vi "ScannedNodeSearch.vi"(6 "Location":T1, 8 "Previously Scanned Nodes":T4 {"Year" format="%02d"; "Patient Number" format="%03d"; "Node Number" format="%02d"}, 9 "Reset Node Count?":bool=TRUE, 10 "Auto Increment":bool, 11 "Searched Node":T2={"Patient Number"=0, "Node Set"="A", "Node Number"=0, "Tissue Type"=enum."Breast", "Tissue Location (Other)"="", "Node Classification"=enum."Whole Node", "Fresh?"=enum."Fresh?", "Year"=0} {"Year" format="%02d"; "Patient Number" format="%03d"; "Node Number" format="%02d"}) -> (3 "Next Node":T2={"Patient Number"=0, "Node Set"="A", "Node Number"=0, "Tissue Type"=enum."Breast", "Tissue Location (Other)"="", "Node Classification"=enum."Whole Node", "Fresh?"=enum."Fresh?", "Year"=0} {"Year" format="%02d"; "Patient Number" format="%03d"; "Node Number" format="%02d"})   [LabVIEW 2022 SP3]
uses:
  ScannedNodeArray.ctl
  LymphNodeInfo.ctl
  TissueTypeScan.ctl
  ScanningControl/-ScanSystem/Controls/location.ctl
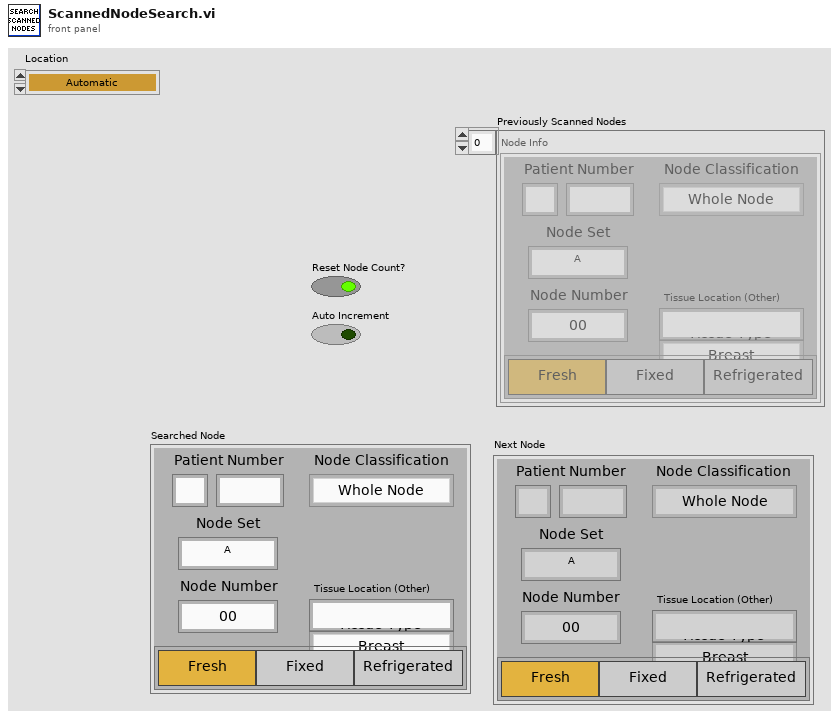
[diagram p1: front panel]
types:
  T1 = typedef "location.ctl" = enum16{"Automatic", "WCM Main", "Hawaii", "Columbia MM3000", "Columbia  NI System", "NYU", "RRI 2", "UHI Allen", "CUMC RT", "Chiba", "Stony Brook", "WCM Microscopy", "WCM Aeoretch", "WCM Optics Lab", "WCM Main 2Axis", "WCM Rotation", "WCM SAM SMAC", "SERI GP"}
  T2 = typedef "LymphNodeInfo.ctl" = cluster{"Patient Number":u32, "Node Set":string, "Node Number":u32, "Tissue Type":T3, "Tissue Location (Other)":string, "Node Classification":enum16{"Whole Node", "Piece A", "Piece B", "Piece C"}, "Fresh?":enum32{"Fresh?", "Fixed?", "Refrigerated?"}, "Year":u32}
  T3 = typedef "TissueTypeScan.ctl" = enum16{"Breast", "Gastric", "Stomach", "Rectal", "Colon", "Head & Neck", "Other"}
  T4 = typedef "ScannedNodeArray.ctl" = T2[]
  T5 = enum16{"Whole Node", "Piece A", "Piece B", "Piece C"}
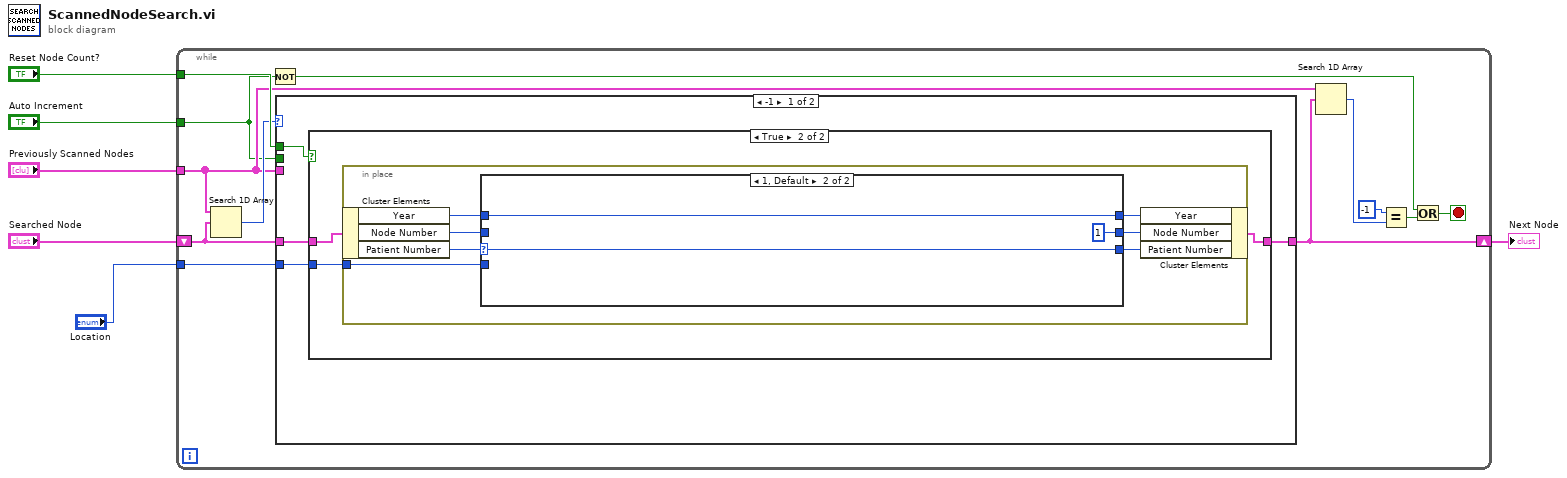
[diagram p0: block diagram]
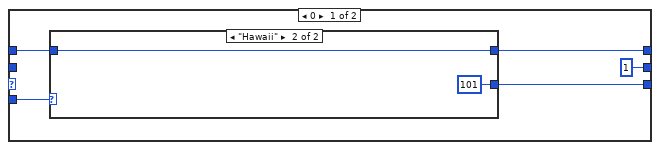
[diagram p3: hidden frame]
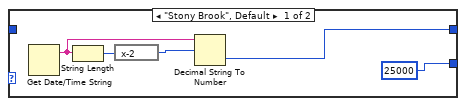
[diagram p4: hidden frame]
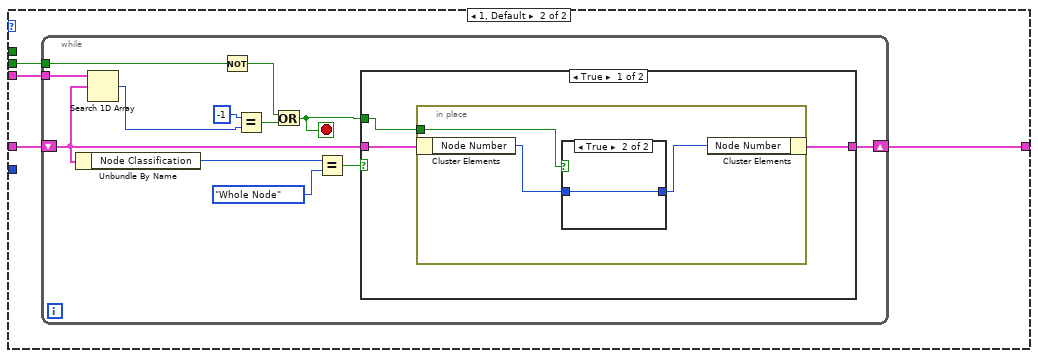
[diagram p5: hidden frame]
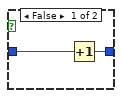
[diagram p6: hidden frame]
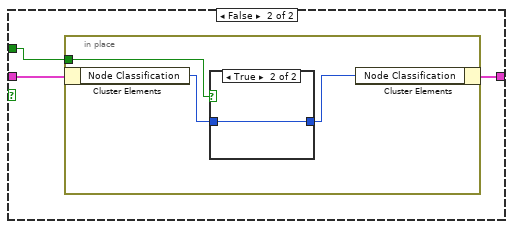
[diagram p7: hidden frame]
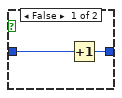
[diagram p8: hidden frame]
diagram:
  n1 = while {
    tunnel: "Reset Node Count?" -> [w17]
    tunnel: "Previously Scanned Nodes" -> [w13]
    tunnel: "Auto Increment" -> [w8]
    shift-right: [w14] -> w6
    shift-left: "Searched Node" -> [w18]
    tunnel: "Location" -> [w7]
    stop <- w9 stop-if-true
    n2 = Search 1D Array(1D array=w13, element=w18) -> (index of element=w15:i32)  [unwired: 1 in]
    n3 = Not(x=w8) -> (.not. x?=w11:bool)
    n4 = case shown="-1" w15 {
      tunnel: [w21 w51] -> w14
      tunnel: w18 -> [w22 w52]
      tunnel: w17 -> [w20 _]
      tunnel: w13 -> [_ w50]
      tunnel: w8 -> [_ w49]
      tunnel: w7 -> [w19 _]
      frame -1 {
        n5 = case shown="True" w20 {
          tunnel: w22 -> [w23 w26]
          tunnel: [w23 w25] -> w21
          tunnel: w19 -> [_ w24]
          frame False {
          }
          frame True {
            n6 = in-place {
              in-place-border: w24 -> [w29]
              n7 = in-place-cluster #1(w26) -> ("Year"=w27:u32, "Node Number"=w30:u32, "Patient Number"=w33:u32)
              n8 = case shown="1, Default" w33 {
                selector: w33 -> [_ w48]
                tunnel: [w38 w48] -> w32
                tunnel: [u32 1 ("Node Number") u32 1 ("Node Number")] -> w31
                tunnel: w30 -> [_ _]
                tunnel: w29 -> [w36 _]
                tunnel: [w35 w46] -> w28
                tunnel: w27 -> [w34 w46]
                frame 0 {
                  n9 = case shown="\"Hawaii\"" w36 {
                    tunnel: [u32 25000 ("y") u32 101] -> w38
                    tunnel: [w39 w44] -> w35
                    tunnel: w34 -> [_ w44]
                    frame "Stony Brook", Default {
                      n10 = Get Date/Time String() -> (date string=w42:string)  [unwired: 3 in, 1 out]
                      n11 = String Length(string=w42) -> (length=w43:i32)
                      n12 = expression code="x-2"(w43) -> (w41:i32)
                      n13 = Decimal String To Number(string=w42, offset=w41) -> (number=w39:i32)  [unwired: 1 in, 1 out]
                    }
                    frame "Hawaii" {
                    }
                  }
                }
                frame 1, Default {
                }
              }
              n14 = in-place-cluster #1("Year"=w28, "Node Number"=w31, "Patient Number"=w32) -> (w25:T2)
            }
          }
        }
      }
      frame 1, Default {
        n15 = while {
          shift-right: [w64] -> w51
          shift-left: w52 -> [w56]
          tunnel: w50 -> [w63]
          tunnel: w49 -> [w59]
          stop <- w57 stop-if-true
          n16 = Unbundle By Name(w56) -> ("Node Classification"=w53:T5)
          n17 = Search 1D Array(1D array=w63, element=w56) -> (index of element=w62:i32)  [unwired: 1 in]
          n18 = Not(x=w59) -> (.not. x?=w58:bool)
          n19 = Equal?(x=-1, y=w62) -> (x = y?=w60:bool)
          n20 = Or(x=w58, y=w60) -> (x .or. y?=w57:bool)
          n21 = Equal?(x=w53, y=T5."Whole Node") -> (x = y?=w55:bool)
          n22 = case shown="True" w55 {
            tunnel: [w67 w76] -> w64
            tunnel: w56 -> [w66 w75]
            tunnel: w57 -> [w65 w74]
            frame True {
              n23 = in-place {
                in-place-border: w65 -> [w68]
                n24 = in-place-cluster #2(w66) -> ("Node Number"=w70:u32)
                n25 = case shown="True" w68 {
                  tunnel: w70 -> [w72 w73]
                  tunnel: [w71 w73] -> w69
                  frame False {
                    n26 = Increment(x=w72) -> (x+1=w71:u32)
                  }
                  frame True {
                  }
                }
                n27 = in-place-cluster #2("Node Number"=w69) -> (w67:T2)
              }
            }
            frame False {
              n28 = in-place {
                in-place-border: w74 -> [w77]
                n29 = in-place-cluster #3(w75) -> ("Node Classification"=w79:T5)
                n30 = case shown="True" w77 {
                  tunnel: w79 -> [w81 w82]
                  tunnel: [w80 w82] -> w78
                  frame False {
                    n31 = Increment(x=w81) -> (x+1=w80:T5)
                  }
                  frame True {
                  }
                }
                n32 = in-place-cluster #3("Node Classification"=w78) -> (w76:T2)
              }
            }
          }
        }
      }
    }
    n33 = Search 1D Array(1D array=w13, element=w14) -> (index of element=w12:i32)  [unwired: 1 in]
    n34 = Equal?(x=-1, y=w12) -> (x = y?=w10:bool)
    n35 = Or(x=w11, y=w10) -> (x .or. y?=w9:bool)
  }
  "Next Node" <- w6
